vi "controlExternalSensor.vi"(7 "Set":bool, 8 "error in":errorcluster, 9 "Enabled":bool, 10 "axis in":u8, 11 "connection ID":refnum<k5>) -> (0 "error out":errorcluster, 1 "Enabled":bool, 2 "axis out":i32, 3 "connection ID":refnum<k5>)   [LabVIEW 2016]
doc: "This function retrieves or sets the sensor source of closed loop to the IDS when enabled."
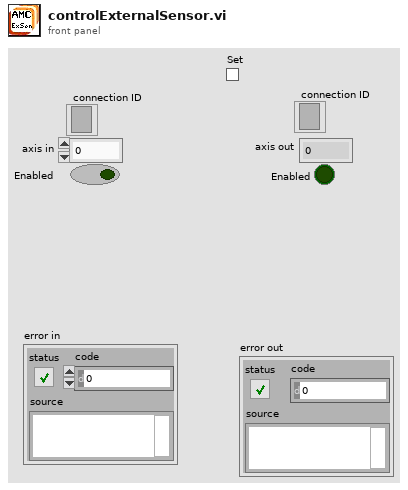
[diagram p1: front panel]
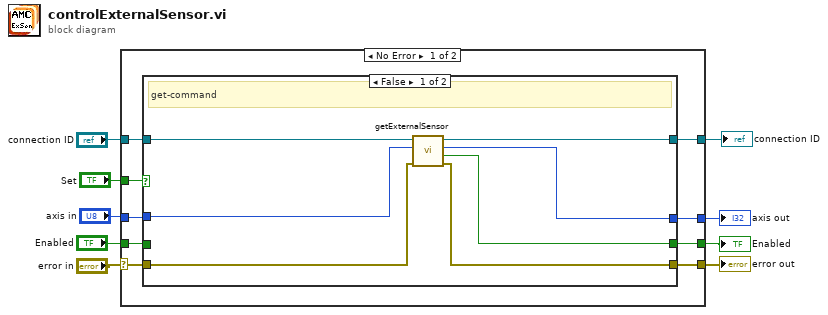
[diagram p0: block diagram]
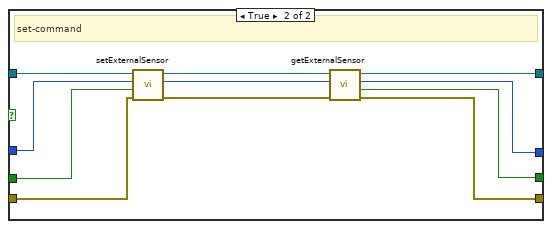
[diagram p2: hidden frame]
diagram:
  n1 = case shown="No Error" "error in" {
    selector: "error in" -> [w14 w40]
    tunnel: "axis in" -> [w18 w37]
    tunnel: [w10 w40] -> w8
    tunnel: "Enabled" -> [w16 w38]
    tunnel: [w13 w38] -> w3
    tunnel: "Set" -> [w15 _]
    tunnel: [w12 w39] -> w6
    tunnel: "connection ID" -> [w17 w39]
    tunnel: [w11 w37] -> w1
    frame No Error {
      n2 = case shown="False" w15 {
        tunnel: w17 -> [w25 w36]
        tunnel: w18 -> [w23 w32]
        tunnel: w16 -> [_ w30]
        tunnel: w14 -> [w21 w31]
        tunnel: [w22 w27] -> w13
        tunnel: [w24 w34] -> w12
        tunnel: [w19 w28] -> w11
        tunnel: [w20 w26] -> w10
        frame False {
          # "get-command"
          n3 = call "getExternalSensor.vi"("error in"=w21, "axis"=w23, "connection ID"=w25) -> ("error out"=w20:errorcluster, "enabled"=w22:bool, "axis_out"=w19:i32, "connection ID"=w24:refnum<k5>)  [unwired: 5 in]
        }
        frame True {
          # "set-command"
          n4 = call "setExternalSensor.vi"("error in"=w31, "enabled"=w30, "axis"=w32, "connection ID"=w36) -> ("error out"=w33:errorcluster, "axis_out"=w29:i32, "connection ID"=w35:refnum<k5>)  [unwired: 5 in]
          n5 = call "getExternalSensor.vi"("error in"=w33, "axis"=w29, "connection ID"=w35) -> ("error out"=w26:errorcluster, "enabled"=w27:bool, "axis_out"=w28:i32, "connection ID"=w34:refnum<k5>)  [unwired: 5 in]
        }
      }
    }
    frame Error {
    }
  }
  "error out" <- w8
  "axis out" <- w1
  "Enabled" <- w3
  "connection ID" <- w6
